vi "Delete Single Attribute.vi"(8 "error in (no error)":errorcluster, 10 "Name":string, 11 "Variant in":refnum<class "Variant.lvclass">) -> (0 "error out":errorcluster, 3 "Variant out":refnum<class "Variant.lvclass">)   [LabVIEW 2020, in "Data.lvlib" / "Variant.lvclass"]
doc: "Delete single attribute from the variant."
uses:
  Variant.lvclass
  Variant.lvclass/Variant.ctl
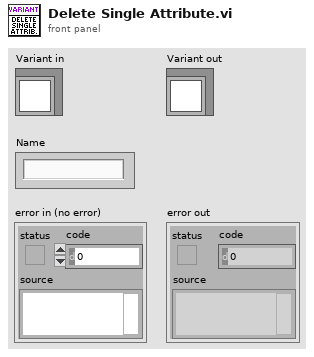
[diagram p1: front panel]
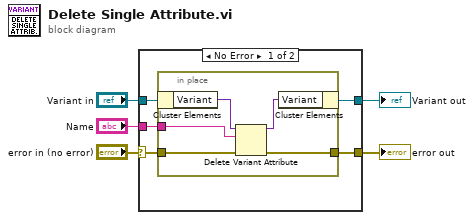
[diagram p0: block diagram]
diagram:
  n1 = case shown="No Error" "error in (no error)" {
    selector: "error in (no error)" -> [w8 w17]
    tunnel: [w7 w17] -> w3
    tunnel: [w9 w16] -> w2
    tunnel: "Variant in" -> [w10 w16]
    tunnel: "Name" -> [w6 _]
    frame No Error {
      n2 = in-place {
        in-place-border: w8 -> [w15]
        in-place-border: [w14] -> w7
        in-place-border: w6 -> [w11]
        n3 = in-place-cluster #1(w10) -> ("Variant"=w12:variant)
        n4 = Delete Variant Attribute(4:w15, 6:w11, 7:w12) -> (0:w14:errorcluster, 3:w13:variant)  [unwired: 1 out]
        n5 = in-place-cluster #1("Variant"=w13) -> (w9:refnum<class "Variant.lvclass">)
      }
    }
    frame Error {
    }
  }
  "error out" <- w3
  "Variant out" <- w2
